vi "FlatToRichcif_channelcore_FIFOInstance.vi"(5 "OutputClusterType":T1, 11 "InputCluster":T2) -> (3 "OutputCluster":T1)   [LabVIEW 2021, in "CIFCoreChannel_server.lvlib"]
uses:
  CIFCoreChannel_server.lvlib
  cif_channelcore_FIFOInstance_Flat.ctl
  cif_channelcore_FIFOInstance.ctl
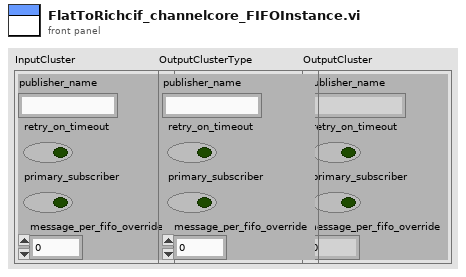
[diagram p1: front panel]
types:
  T1 = typedef "CIFCoreChannel_server.lvlib/cif_channelcore_FIFOInstance.ctl" = cluster{"publisher_name":string, "retry_on_timeout":bool, "primary_subscriber":bool, "message_per_fifo_override":u32}
  T2 = typedef "CIFCoreChannel_server.lvlib/cif_channelcore_FIFOInstance_Flat.ctl" = cluster{"publisher_name":string, "retry_on_timeout":bool, "primary_subscriber":bool, "message_per_fifo_override":u32}
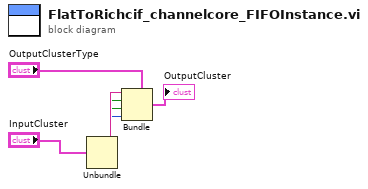
[diagram p0: block diagram]
diagram:
  n1 = Unbundle "Unbundle"("InputCluster") -> ("publisher_name"=w4:string, "retry_on_timeout"=w3:bool, "primary_subscriber"=w2:bool, "message_per_fifo_override"=w1:u32)
  n2 = Bundle "Bundle"(cluster="OutputClusterType", "publisher_name"=w4, "retry_on_timeout"=w3, "primary_subscriber"=w2, "message_per_fifo_override"=w1) -> (→"OutputCluster":T1)
